vi "Read Pressure.vi"(0 "Session Handle in":T2, 5 "Pressure Sensor":T1=224 items=["PS1"=224, "PS2"=225], 11 "error in (no error)":errorcluster) -> (4 "Session Handle out":T2, 6 "Pressure":dbl, 15 "error out":errorcluster)   [LabVIEW 2015, in "Gas.lvclass"]
uses:
  Gas.lvclass
  Typedefs/Session Handle.ctl
  Typedefs/Pressure Sensor.ctl
panel:
  out "Success?":bool
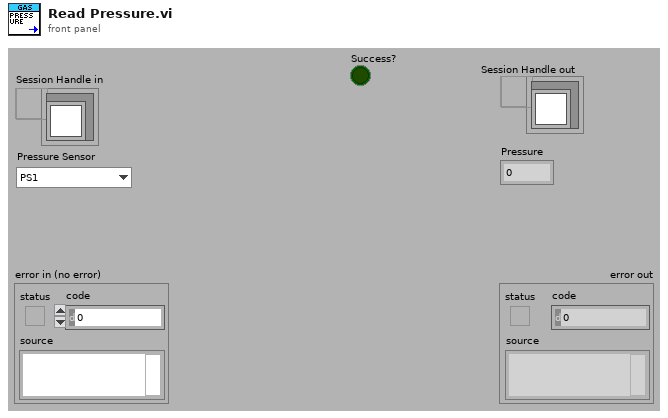
[diagram p1: front panel]
types:
  T1 = typedef "Gas.lvclass/Pressure Sensor.ctl" = u16
  T2 = typedef "Gas.lvclass/Session Handle.ctl" = refnum<data-value>
  T3 = typedef "XNET Frame CAN.ctl" = cluster{"timestamp":timestamp, "payload":u8[], "identifier":u32, "type":T4, "extended?":bool, "echo?":bool}
  T4 = typedef "XNET Frame Type CAN.ctl" = u8
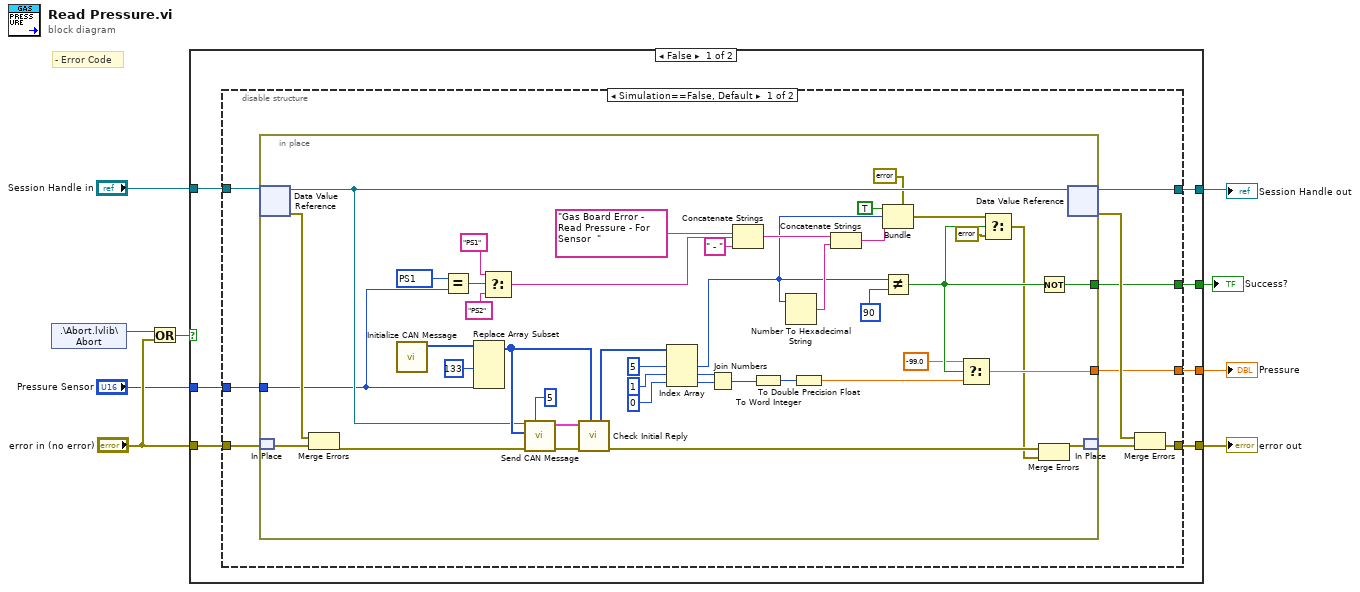
[diagram p0: block diagram]
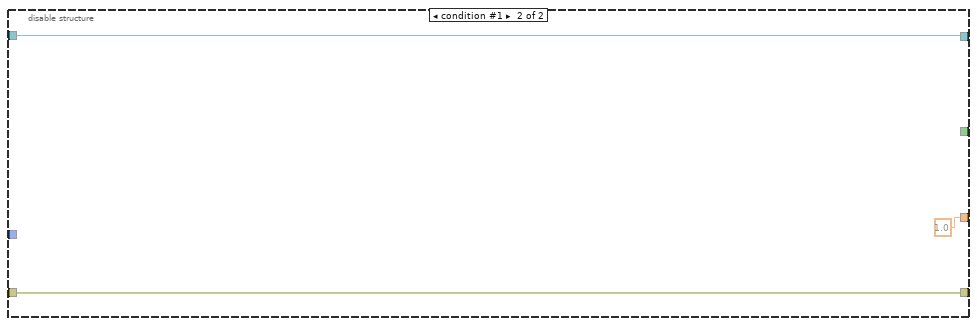
[diagram p2: hidden frame]
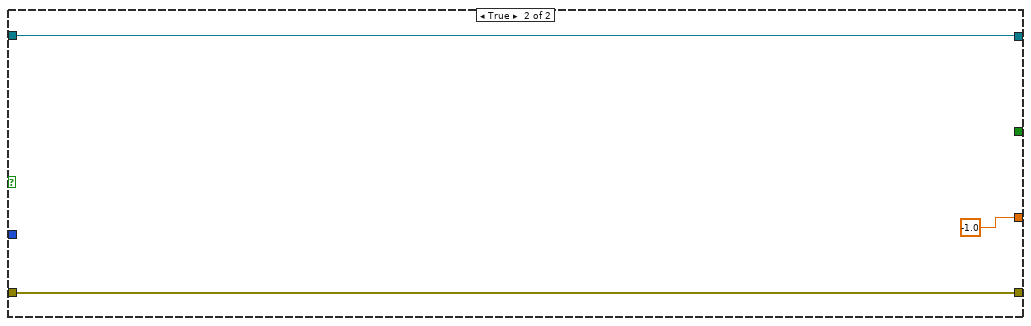
[diagram p3: hidden frame]
diagram:
  # "- Error Code"
  n1 = shared-variable ".\\Abort.lvlib\\Abort"() -> (w6:bool)  [unwired: 1 in, 1 out]
  n2 = Or(x=w6, y="error in (no error)") -> (x .or. y?=w4:bool)
  n3 = case shown="False" w4 {
    tunnel: [w16 w74] -> w8
    tunnel: [w15 w73] -> w7
    tunnel: "Session Handle in" -> [w14 w74]
    tunnel: "error in (no error)" -> [w13 w73]
    tunnel: [w12 -1.0] -> w3
    tunnel: [w11 _] -> w2
    tunnel: "Pressure Sensor" -> [w10 _]
    frame False {
      n4 = disable-structure shown="Simulation==False, Default" {
        disable-tunnel: [w25 w71] -> w16
        disable-tunnel: [w22 w70] -> w15
        disable-tunnel: w14 -> [w21 w71]
        disable-tunnel: w13 -> [w20 w70]
        disable-tunnel: [w19 1.0] -> w12
        disable-tunnel: [w18 _] -> w11
        disable-tunnel: w10 -> [w17 _]
        frame condition #0 (active) {
          n5 = in-place {
            in-place-border: [w34] -> w19
            in-place-border: [w54] -> w18
            in-place-border: w17 -> [w46]
            w45 = T1 224 items=["PS1"=224, "PS2"=225] ("Pressure Sensor")
            n6 = in-place-dvr #1(w21) -> (w59:refnum<class "Gas.lvclass">, w64:errorcluster)
            n7 = in-place-match #2(w20) -> (w63:errorcluster)
            n8 = Merge Errors(w64, w63) -> (w58:errorcluster)
            n9 = call "Initialize CAN Message.vi"() -> ("Initial Payload"=w66:u8[])  [unwired: 11 in]
            n10 = Equal?(x=w45, y=w46) -> (x = y?=w44:bool)
            n11 = Replace Array Subset(array=w66, new element #1=u8 133 ("new element/subarray"), new element #2=w46) -> (w62:u8[])  [unwired: 2 in]
            n12 = Select(t="PS1", s=w44, f="PS2") -> (s? t:f=w40:string)
            n13 = call "Send CAN Message.vi"("Number of Retries"=5, "error in (no error)"=w58, "payload"=w62, "Gas In"=w59) -> ("error out"=w33:errorcluster, "Reply"=w60:T3[])  [unwired: 5 in, 1 out]
            n14 = call "Check Initial Reply.vi"("Write Message"=w62, "error in (no error)"=w33, "Reply"=w60) -> ("error out"=w32:errorcluster, "Data Packet"=w65:u8[])  [unwired: 5 in, 2 out]
            n15 = Index Array(array=w65, index #1=5 ("index"), index #2=1 ("index"), index #3=0 ("index")) -> (element #1=w27:u8, element #2=w50:u8, element #3=w49:u8)
            n16 = Join Numbers(hi=w50, lo=w49) -> ((hi.lo)=w48:u16)
            n17 = Concatenate Strings("Gas Board Error -  Read Pressure - For Sensor  " ("string"), w40, " - ") -> (w38:string)
            n18 = To Word Integer(number=w48) -> (16bit integer=w51:i16)
            n19 = Number To Hexadecimal String(2:w27) -> (0:w57:string)  [unwired: 1 in]
            n20 = To Double Precision Float(number=w51) -> (double precision float=w36:dbl)
            n21 = Concatenate Strings(w38, w57) -> (w28:string)
            n22 = Bundle(cluster=errorcluster {"status"=FALSE, "code"=0, "source"=""} ("f"), "status"=TRUE, "code"=w27, "source"=w28) -> (w26:errorcluster)
            n23 = Not Equal?(x=w27, y=u8 90 ("new element/subarray")) -> (x != y?=w37:bool)
            n24 = Select(t=-99.0, s=w37, f=w36) -> (s? t:f=w34:dbl)
            n25 = Select(t=w26, s=w37, f=errorcluster {"status"=FALSE, "code"=0, "source"=""}) -> (s? t:f=w31:errorcluster)
            n26 = Not(x=w37) -> (.not. x?=w54:bool)
            n27 = Merge Errors(w32, w31) -> (w67:errorcluster)
            n28 = in-place-dvr #1(w59) -> (w25:T2, w23:errorcluster)
            n29 = in-place-match #2(w67) -> (w24:errorcluster)
          }
          n30 = Merge Errors(w23, w24) -> (w22:errorcluster)
        }
        frame condition #1 {
        }
      }
    }
    frame True {
    }
  }
  "Session Handle out" <- w8
  "error out" <- w7
  "Pressure" <- w3
  "Success?" <- w2
